vi "OutputShooter.vi"() -> ()   [LabVIEW 2020]
doc: "Runs feedback and feedforward control loops, manages safety interlocks, and sends commands to actuators specific to the shooter subsystem, specifically the lower shooter Falcon 500, the upper shooter Falcon 500, and the cowl Falcon 500."
uses:
  <vilib>/Rock Robotics/WPI/ThirdParty/Phoenix-LabVIEW/Motor Controller/Controls/CTRE_Phoenix_MotorControl_ControlMode.ctl
  60a0c6b8-2381-40aa-8ec2-a2ed4196b17e.vi
  0f04a1d6-f6ee-4c5b-8505-751c5889a14e.vi
  ceb5ace5-ff86-47da-bc92-28042f34dd1c.vi
  refnumbers.vi
  GRNF_CTREMotor.vi
  <vilib>/Rock Robotics/WPI/ThirdParty/Phoenix-LabVIEW/Motor Controller/Get/CTRE_Phoenix_MotorController_GetGeneralStatus.vi
  sensordata.vi
  robotconstants.vi
  robotoutputs.vi
  driverdata.vi
  drivercommands.vi
  TAI_Motor.vi
  <vilib>/Rock Robotics/WPI/ThirdParty/Phoenix-LabVIEW/Motor Controller/Get/CTRE_Phoenix_MotorController_GetSelectedSensorData.vi
  <vilib>/Rock Robotics/WPI/ThirdParty/Phoenix-LabVIEW/Motor Controller/Get/CTRE_Phoenix_MotorController_GetVoltage.vi
panel:
  in  "Shooter Upper PID Configuration":T1={"P Gain"=0.006, "I Gain"=0.0, "D Gain"=0.0, "F Gain"=0.2, "I Zone"=200.0} {"I Zone" step=0.01; "F Gain" step=0.01; "D Gain" step=0.01; "I Gain" step=0.01; "P Gain" min=0.0 step=0.01}
  out "Cowl Velocity":cluster{dbl}(graph)
  in  "Cowl PID Parameters":T2={"Kp"=0.03, "Ki"=0.0, "Kd"=0.0, "Kf (don't use)"=0.0, "I-Zone"=10.0} {"Kd" min=0.0; "Ki" min=0.0; "Kp" min=0.0}
  in  "Arbitrary Feed Forward [-1,1]":dbl=0.03
  in  "Cowl S-Curve Strength":i32=4
  in  "Cowl Acceleration (deg/s^2)":dbl=300.0
  in  "Cowl Cruise Velocity (deg/s)":dbl=60.0
  out "Cowl Position":cluster{dbl, "Interlock Output":dbl}(graph)
  out "Position":dbl
  in  "Plot Cowl":bool
  in  "Manual Override Cowl":bool
  in  "Manual Cowl Command (deg)":dbl
  in  "Manual Shooter Upper Speed Ratio":dbl=1.5 min=0.0 max=6000.0 step=100.0
  in  "Manual Shooter Speed Goal (rpm)":dbl min=0.0 max=6000.0 step=100.0
  in  "Override Shooter State Controller":bool
  out "Shooter Upper":T3(graph)
  in  "Plot Shooter":bool
  out "Shooter Lower":T3(graph)
  in  "Shooter Lower PID Configuration":T1={"P Gain"=0.005, "I Gain"=0.0, "D Gain"=0.0, "F Gain"=0.2, "I Zone"=200.0} {"I Zone" step=0.01; "F Gain" step=0.01; "D Gain" step=0.01; "I Gain" step=0.01; "P Gain" min=0.0 step=0.01}
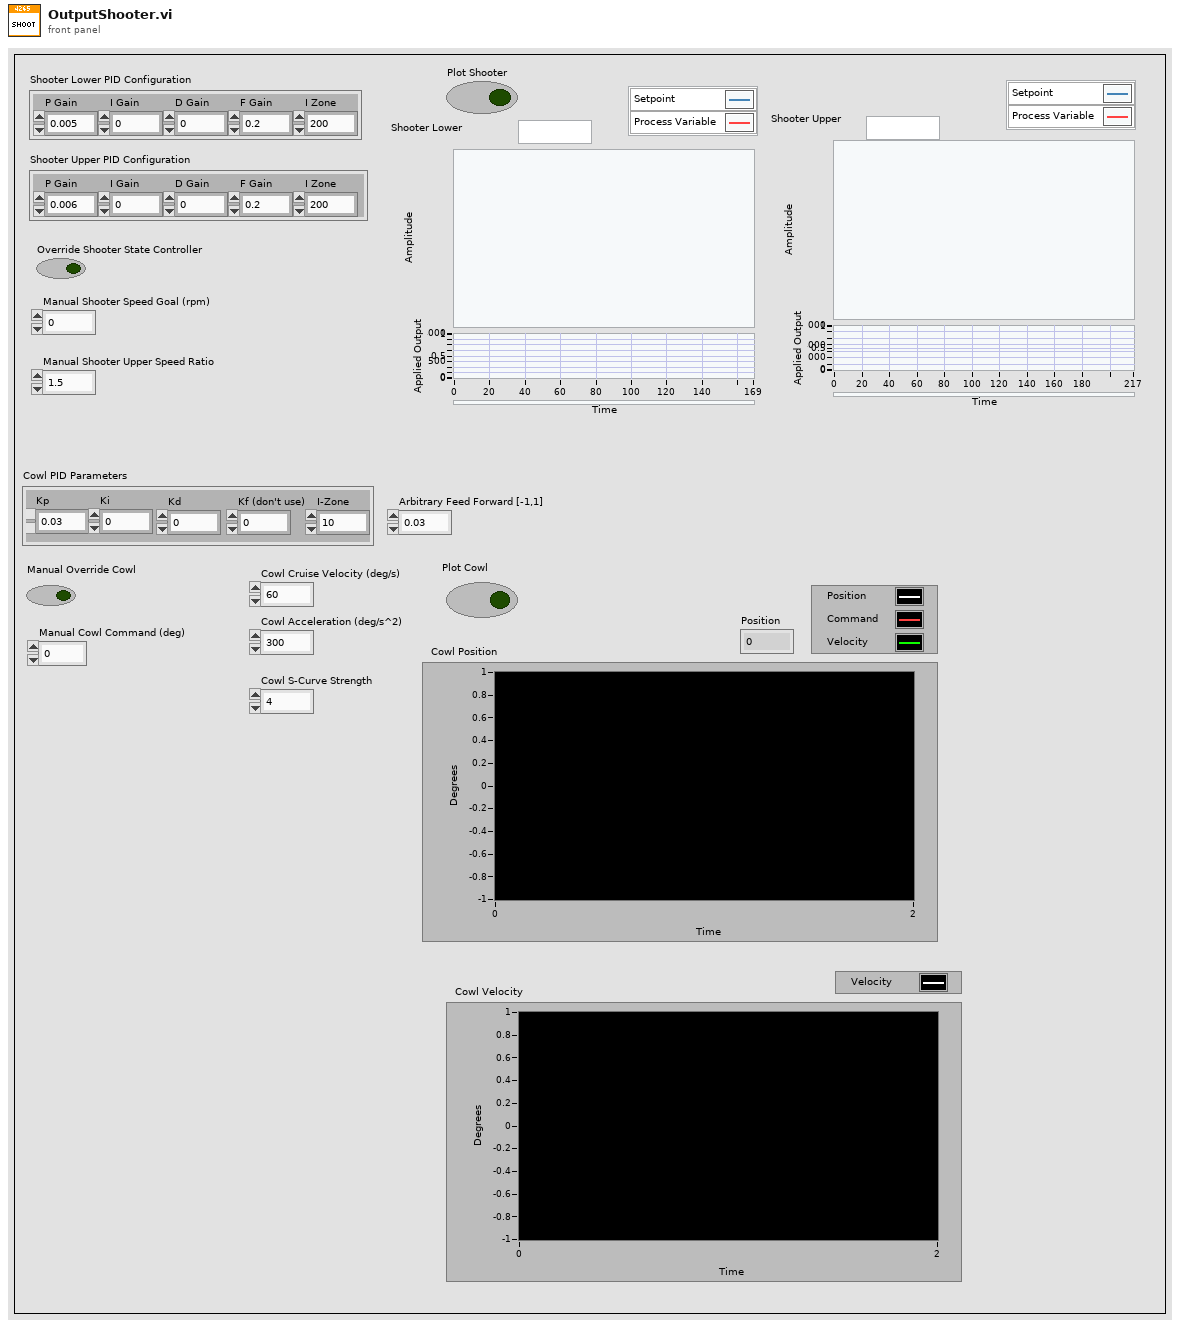
[diagram p1: front panel]
types:
  T1 = cluster{"P Gain":dbl, "I Gain":dbl, "D Gain":dbl, "F Gain":dbl, "I Zone":dbl}
  T2 = cluster{"Kp":dbl, "Ki":dbl, "Kd":dbl, "Kf (don't use)":dbl, "I-Zone":dbl}
  T3 = cluster{"Sensor Velocity":dbl, "Setpoint":dbl, "Applied Output":dbl}
  T4 = cluster{"Cowl Cruise Velocity (deg/s)":i32, "Cowl Acceleration (deg/s^2)":i32, "Cowl S-Curve Strength":i32}
  T5 = typedef "WPI_MotorControlDeviceRef.ctl" = cluster{"DeviceStatus":errorcluster, "Type":T6, "PWM":cluster{"PWM Channel":T7, "DeadBand":T8}, "CAN":cluster{"Device Number":u8, "SetOutput VI Ref":variant, "GetOutput VI Ref":variant, "Enable VI Ref":variant, "Disable VI Ref":variant, "Data":variant}, "Invert":bool, "DIO PWM":cluster{"PWM \"Enable\" Channel":T7, "DIOChannel":T9, "PWM Rate":dbl}}
  T6 = typedef "WPI_MotorControlType.ctl" = enum16{"PWM", "CAN", "DIO PWM"}
  T7 = typedef "FPGA_DIOPWMChannel.ctl" = enum8{"PWM 0", "PWM 1", "PWM 2", "PWM 3", "PWM 4", "PWM 5", "PWM 6", "PWM 7", "PWM 8", "PWM 9", "PWM MXP 0", "PWM MXP 1", "PWM MXP 2", "PWM MXP 3", "PWM MXP 4", "PWM MXP 5", "PWM MXP 6", "PWM MXP 7", "PWM MXP 8", "PWM MXP 9", "Invalid"}
  T8 = typedef "WPI_PWMDeadband.ctl" = cluster{"Name":string, "maxPositivePwm":i32, "minPositivePwm":i32, "centerPwm":i32, "maxNegativePwm":i32, "minNegativePwm":i32, "angularRange":u16}
  T9 = typedef "FPGA_DIOChannel.ctl" = enum8{"DIO 0", "DIO 1", "DIO 2", "DIO 3", "DIO 4", "DIO 5", "DIO 6", "DIO 7", "DIO 8", "DIO 9", "DIO MXP 0", "DIO MXP 1", "DIO MXP 2", "DIO MXP 3", "DIO MXP 4", "DIO MXP 5", "DIO MXP 6", "DIO MXP 7", "DIO MXP 8", "DIO MXP 9", "DIO MXP 10", "DIO MXP 11", "DIO MXP 12", "DIO MXP 13", "DIO MXP 14", "DIO MXP 15", "SPI Port CS1", "SPI Port CS2", "SPI Port CS3", "SPI Port MISO", "SPI Port MOSI", "Invalid"}
  T10 = cluster{"P Gain":bool, "I Gain":bool, "D Gain":bool, "F Gain":bool, "I Zone":bool}
  T11 = cluster{"Cowl Cruise Velocity (deg/s)":bool, "Cowl Acceleration (deg/s^2)":bool, "Cowl S-Curve Strength":bool}
  T12 = enum16{"No Changed Output", "New Normal Output", "New Testing Output"}
  T13 = cluster{"Kp":bool, "Ki":bool, "Kd":bool, "Kf (don't use)":bool, "I-Zone":bool}
  T14 = typedef "CTRE_Phoenix_MotorControl_ControlMode.ctl" = u16
  T15 = cluster{"Interlocked Output":dbl, dbl, "Percent Output":dbl}
  T16 = enum16{"DemandType_Neutral", "DemandType_AuxPID", "DemandType_ArbitraryFeedForward"}
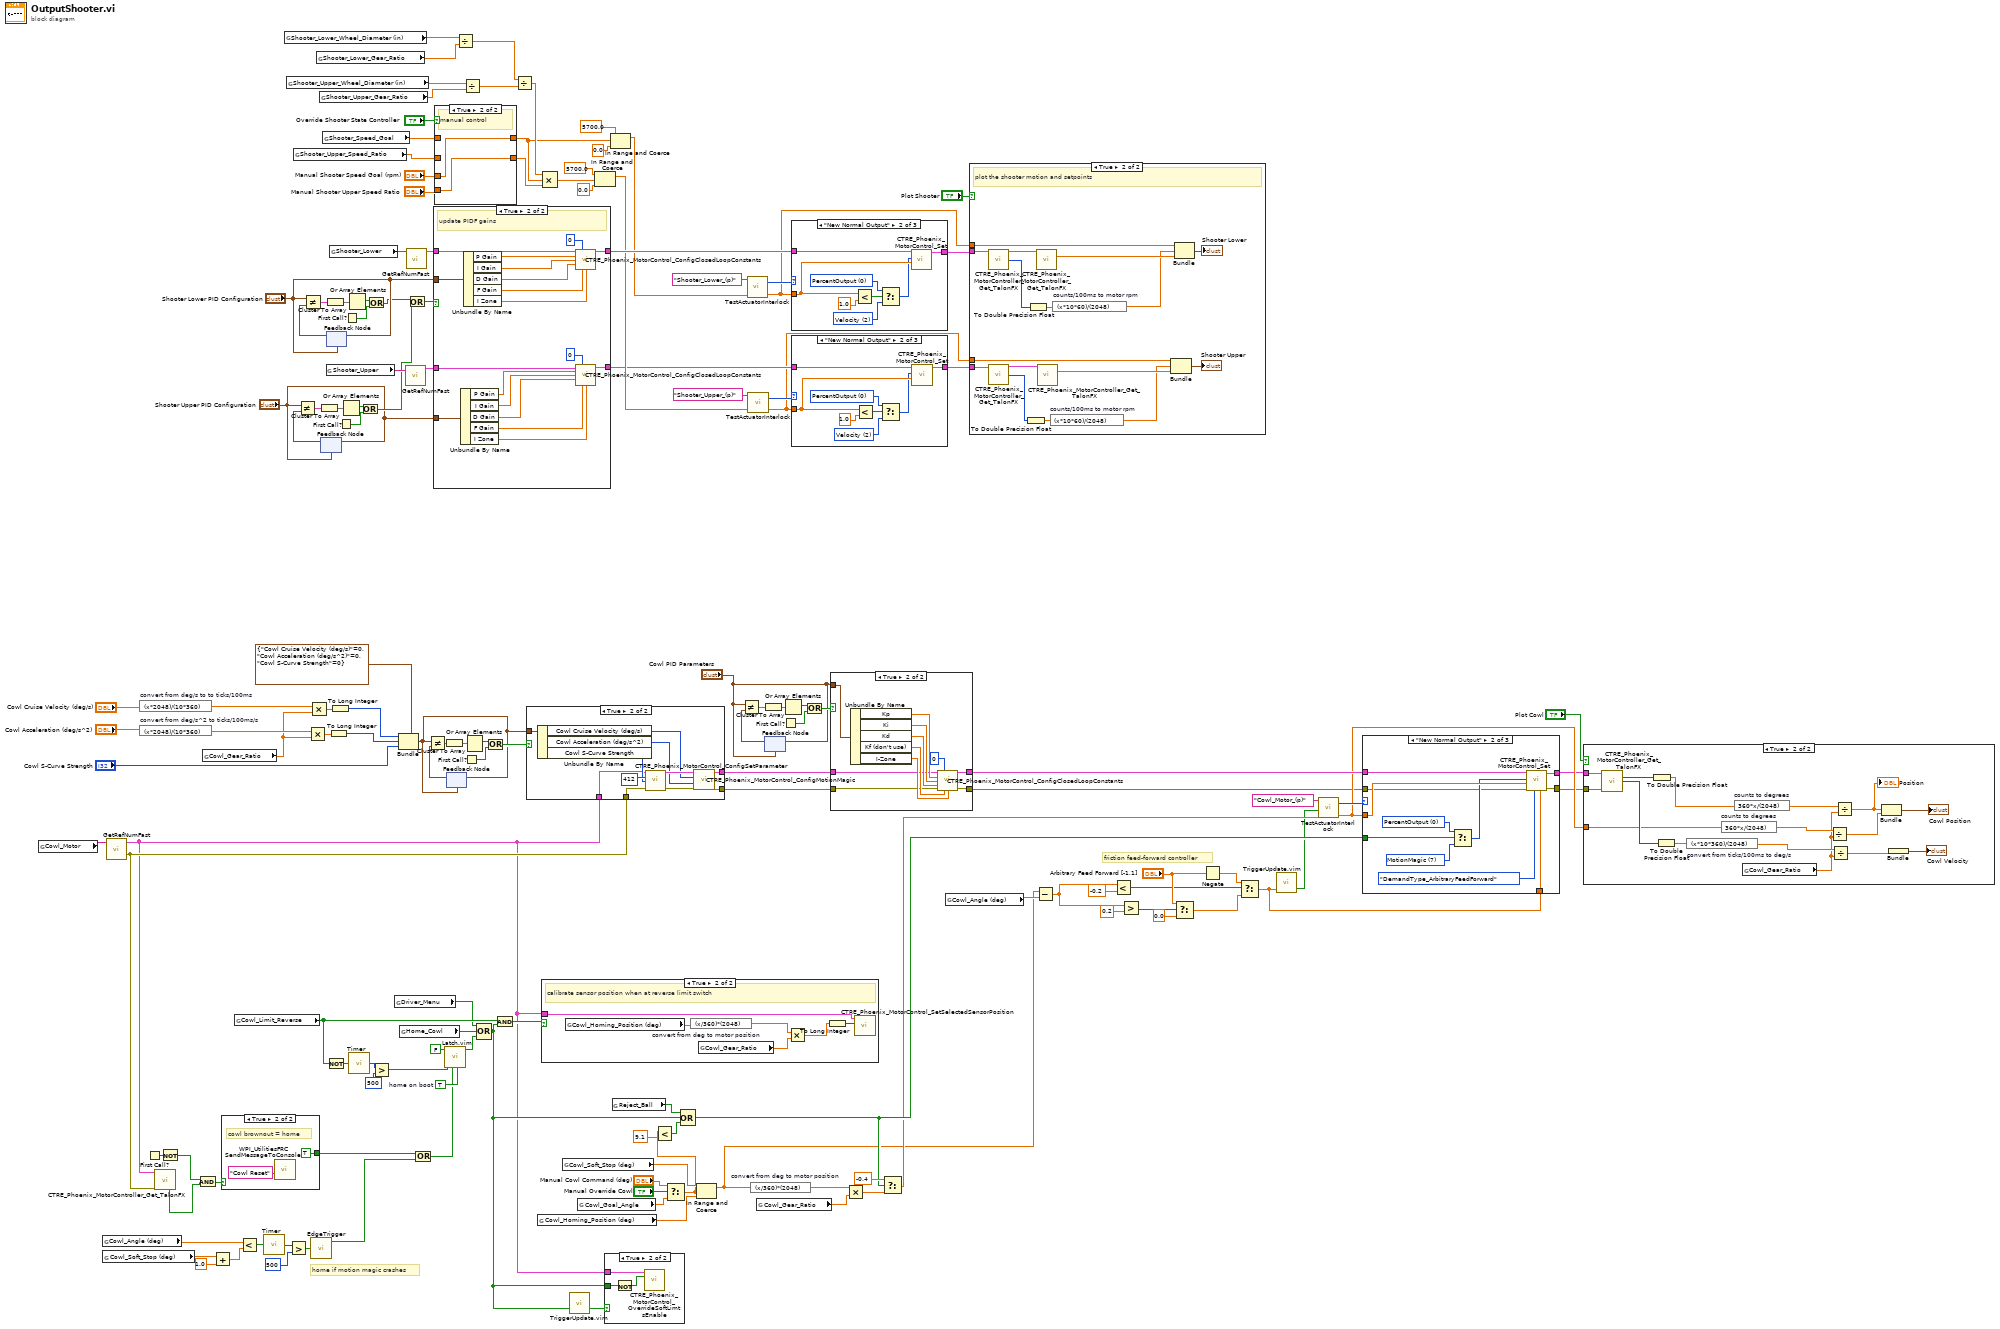
[diagram p0: block diagram]
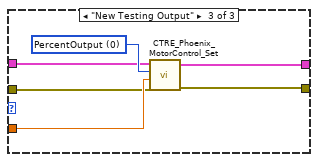
[diagram p4: hidden frame]
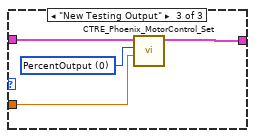
[diagram p6: hidden frame]
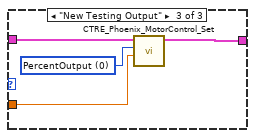
[diagram p8: hidden frame]
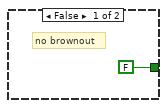
[diagram p9: hidden frame]
diagram:
  w29 = TRUE  # home on boot
  # "home if motion magic crashes"
  # "friction feed-forward controller"
  n1 = global read "refnumbers.vi" "Cowl_Motor"() -> (w129:string)
  n2 = global read "sensordata.vi" "Cowl_Angle (deg)"() -> (w7:dbl)
  n3 = global read "robotconstants.vi" "Cowl_Soft_Stop (deg)"() -> (w12:dbl)
  n4 = call-poly "GetRefNumFast.vi"("RefNum Name"=w129) -> ("Error"=w77:errorcluster, "Device Reference"=w9:T5)  [unwired: 5 in]
  n5 = expression code="(x*2048)/(10*360)" "convert from deg/s to to ticks/100ms"("Cowl Cruise Velocity (deg/s)") -> (w70:dbl)
  n6 = expression code="(x*2048)/(10*360)" "convert from deg/s^2 to ticks/100ms/s"("Cowl Acceleration (deg/s^2)") -> (w71:dbl)
  n7 = First Call?() -> (First Call?: T/F=w99:bool)
  n8 = call-poly <vilib>:"CTRE_Phoenix_MotorController_Get_TalonFX.vi"("PhoenixMotorControlDevRef"=w9, "error in"=w77) -> ("Has Reset Occurred?"=w97:bool)  [unwired: 8 in, 5 out]
  n9 = Not(x=w99) -> (.not. x?=w98:bool)
  n10 = And(x=w98, y=w97) -> (x .and. y?=w100:bool)
  n11 = global read "robotconstants.vi" "Cowl_Gear_Ratio"() -> (w69:dbl)
  n12 = Add(x=w12, y=1.0) -> (x+y=w6:dbl)
  n13 = case shown="True" w100 {
    tunnel: [FALSE TRUE] -> w16
    frame False {
      # "no brownout"
    }
    frame True {
      # "cowl brownout = home"
      n14 = call <vilib>:"WPI_UtilitiesFRC SendMessageToConsole.vi"("Message"="Cowl Reset") -> ()  [unwired: 14 in, 1 out]
    }
  }
  n15 = global read "sensordata.vi" "Cowl_Limit_Reverse"() -> (w26:bool)
  n16 = Less?(x=w7, y=w6) -> (x < y?=w5:bool)
  n17 = call "Timer.vi"("Reset Timer"=w5) -> ("Time (ms)"=w17:u32)
  n18 = global read "robotconstants.vi" "Shooter_Lower_Wheel_Diameter (in)"() -> (w40:dbl)
  n19 = global read "robotconstants.vi" "Shooter_Upper_Wheel_Diameter (in)"() -> (w37:dbl)
  n20 = Greater?(x=w17, y=u32 500) -> (0:w14:bool)
  n21 = global read "robotoutputs.vi" "Shooter_Upper_Speed_Ratio"() -> (w107:dbl)
  n22 = Multiply(x=w71, y=w69) -> (x*y=w72:dbl)
  n23 = Multiply(x=w70, y=w69) -> (x*y=w73:dbl)
  n24 = call "EdgeTrigger.vi"("Input Signal"=w14) -> ("Rising Edge Trigger"=w13:bool)  [unwired: 2 out]
  n25 = global read "robotconstants.vi" "Shooter_Lower_Gear_Ratio"() -> (w39:dbl)
  n26 = global read "robotconstants.vi" "Shooter_Upper_Gear_Ratio"() -> (w36:dbl)
  n27 = feedback #1("Shooter Upper PID Configuration") -> (w45:T1)
  n28 = Not Equal?(x="Shooter Upper PID Configuration", y=w45) -> (x != y?=w47:T10)
  n29 = Cluster To Array(cluster=w47) -> (array=w46:bool[])
  n30 = feedback-in #1("Shooter Upper PID Configuration") -> ()
  n31 = global read "robotoutputs.vi" "Shooter_Speed_Goal"() -> (w108:dbl)
  n32 = global read "refnumbers.vi" "Shooter_Upper"() -> (w135:string)
  n33 = Not(x=w26) -> (.not. x?=w28:bool)
  n34 = feedback #2("Shooter Lower PID Configuration") -> (w141:T1)
  n35 = Not Equal?(x="Shooter Lower PID Configuration", y=w141) -> (x != y?=w143:T10)
  n36 = Cluster To Array(cluster=w143) -> (array=w142:bool[])
  n37 = feedback-in #2("Shooter Lower PID Configuration") -> ()
  n38 = To Long Integer(number=w72) -> (32bit integer=w64:i32)
  n39 = global read "refnumbers.vi" "Shooter_Lower"() -> (w136:string)
  n40 = To Long Integer(number=w73) -> (32bit integer=w65:i32)
  n41 = First Call?() -> (First Call?: T/F=w49:bool)
  n42 = Or Array Elements(Boolean array=w46) -> (logical OR=w48:bool)
  n43 = First Call?() -> (First Call?: T/F=w145:bool)
  n44 = Or Array Elements(Boolean array=w142) -> (logical OR=w144:bool)
  n45 = call "Timer.vi"("Reset Timer"=w28) -> ("Time (ms)"=w32:u32)
  n46 = Or(x=w48, y=w49) -> (x .or. y?=w42:bool)
  n47 = Or(x=w144, y=w145) -> (x .or. y?=w43:bool)
  n48 = Greater?(x=w32, y=u32 500) -> (0:w27:bool)
  n49 = global read "drivercommands.vi" "Driver_Menu"() -> (w1:bool)
  n50 = Bundle(cluster=T4 {"Cowl Cruise Velocity (deg/s)"=0, "Cowl Acceleration (deg/s^2)"=0, "Cowl S-Curve Strength"=0}, "Cowl Cruise Velocity (deg/s)"=w65, "Cowl Acceleration (deg/s^2)"=w64, "Cowl S-Curve Strength"="Cowl S-Curve Strength") -> (w110:T4)
  n51 = global read "driverdata.vi" "Home_Cowl"() -> (w22:bool)
  n52 = call-poly "GetRefNumFast.vi"("RefNum Name"=w135) -> ("Device Reference"=w138:T5)  [unwired: 5 in, 1 out]
  n53 = call-poly "GetRefNumFast.vi"("RefNum Name"=w136) -> ("Device Reference"=w140:T5)  [unwired: 5 in, 1 out]
  n54 = Or(x=w43, y=w42) -> (x .or. y?=w44:bool)
  n55 = Compound Arithmetic op=OR(w16, w13) -> (w15:bool)
  n56 = case shown="True" w44 {
    tunnel: w140 -> [w150 w167]
    tunnel: "Shooter Lower PID Configuration" -> [_ w166]
    tunnel: [w150 w168] -> w94
    tunnel: [w149 w165] -> w87
    tunnel: w138 -> [w149 w164]
    tunnel: "Shooter Upper PID Configuration" -> [_ w156]
    frame False {
      # "do not update PIDF gains"
    }
    frame True {
      # "update PIDF gains"
      n57 = Unbundle By Name(w156) -> ("P Gain"=w155:dbl, "I Gain"=w154:dbl, "D Gain"=w153:dbl, "F Gain"=w152:dbl, "I Zone"=w151:dbl)
      n58 = Unbundle By Name(w166) -> ("P Gain"=w163:dbl, "I Gain"=w162:dbl, "D Gain"=w161:dbl, "F Gain"=w157:dbl, "I Zone"=w160:dbl)
      n59 = call <vilib>:"CTRE_Phoenix_MotorControl_ConfigClosedLoopConstants.vi"("PhoenixMotorControlDevRef"=w167, "slotIdx"=0, "P"=w163, "I"=w162, "D"=w161, "F"=w157, "I Zone"=w160) -> ("PhoenixMotorControlDevRef"=w168:T5)  [unwired: 7 in, 1 out]
      n60 = call <vilib>:"CTRE_Phoenix_MotorControl_ConfigClosedLoopConstants.vi"("PhoenixMotorControlDevRef"=w164, "slotIdx"=0, "P"=w155, "I"=w154, "D"=w153, "F"=w152, "I Zone"=w151) -> ("PhoenixMotorControlDevRef"=w165:T5)  [unwired: 7 in, 1 out]
    }
  }
  n61 = case shown="True" "Override Shooter State Controller" {
    tunnel: "Manual Shooter Speed Goal (rpm)" -> [_ w172]
    tunnel: "Manual Shooter Upper Speed Ratio" -> [_ w171]
    tunnel: w107 -> [w169 _]
    tunnel: w108 -> [w170 _]
    tunnel: [w170 w172] -> w104
    tunnel: [w169 w171] -> w131
    frame False {
      # "state controller"
    }
    frame True {
      # "manual control"
    }
  }
  n62 = call "Latch.vim"("Default Value"=w29, "Reset"=w15, "Latch Signal"=w27, "Latch Value"=FALSE) -> ("Latched"=w25:bool)  [unwired: 7 in]
  n63 = feedback #3(w110) -> (w111:T4)
  n64 = Not Equal?(x=w110, y=w111) -> (x != y?=w114:T11)
  n65 = Cluster To Array(cluster=w114) -> (array=w113:bool[])
  n66 = feedback-in #3(w110) -> ()
  n67 = Divide(x=w40, y=w39) -> (x/y=w38:dbl)
  n68 = First Call?() -> (First Call?: T/F=w116:bool)
  n69 = Divide(x=w37, y=w36) -> (x/y=w35:dbl)
  n70 = Or Array Elements(Boolean array=w113) -> (logical OR=w115:bool)
  n71 = Compound Arithmetic op=OR(w1, w22, w25) -> (w10:bool)
  n72 = Or(x=w115, y=w116) -> (x .or. y?=w112:bool)
  n73 = And(x=w26, y=w10) -> (x .and. y?=w23:bool)
  n74 = Divide(x=w38, y=w35) -> (x/y=w130:dbl)
  n75 = case shown="True" w112 {
    tunnel: w110 -> [_ w182]
    tunnel: w9 -> [w174 w178]
    tunnel: w77 -> [w173 w177]
    tunnel: [w174 w176] -> w84
    tunnel: [w173 w175] -> w83
    frame False {
    }
    frame True {
      n76 = Unbundle By Name(w182) -> ("Cowl Cruise Velocity (deg/s)"=w179:i32, "Cowl Acceleration (deg/s^2)"=w180:i32, "Cowl S-Curve Strength"=w181:i32)
      n77 = call <vilib>:"CTRE_Phoenix_MotorControl_ConfigSetParameter.vi"("PhoenixMotorControlDevRef"=w178, "Parameter"=412 ("New Sensor Position"), "value"=w181, "error in (no error)"=w177) -> ("PhoenixMotorControlDevRef"=w184:T5, "error out"=w183:errorcluster)  [unwired: 10 in]
      n78 = call <vilib>:"CTRE_Phoenix_MotorControl_ConfigMotionMagic.vi"("error in (no error)"=w183, "Acceleration"=w180, "Cruise Velocity"=w179, "PhoenixMotorControlDevRef"=w184) -> ("error out"=w175:errorcluster, "PhoenixMotorControlDevRef"=w176:T5)  [unwired: 6 in]
    }
  }
  n79 = global read "robotconstants.vi" "Cowl_Homing_Position (deg)"() -> (w19:dbl)
  n80 = case shown="True" w23 {
    tunnel: w9 -> [_ w190]
    frame False {
    }
    frame True {
      # "calibrate sensor position when at reverse limit switch"
      n81 = global read "robotconstants.vi" "Cowl_Homing_Position (deg)"() -> (w189:dbl)
      n82 = expression code="(x/360)*(2048)" "convert from deg to motor position"(w189) -> (w187:dbl)
      n83 = global read "robotconstants.vi" "Cowl_Gear_Ratio"() -> (w188:dbl)
      n84 = Multiply(x=w187, y=w188) -> (x*y=w186:dbl)
      n85 = To Long Integer(number=w186) -> (32bit integer=w191:i32)
      n86 = call <vilib>:"CTRE_Phoenix_MotorControl_SetSelectedSensorPosition.vi"("New Sensor Position"=w191, "PhoenixMotorControlDevRef"=w190) -> ()  [unwired: 8 in, 2 out]
    }
  }
  n87 = Compound Arithmetic op=MULTIPLY(w130, w104, w131) -> (w101:dbl)
  n88 = global read "robotconstants.vi" "Cowl_Soft_Stop (deg)"() -> (w52:dbl)
  n89 = call "TriggerUpdate.vim"("Trigger"=w10) -> ("Update"=w11:bool)  [unwired: 2 in]
  n90 = global read "robotoutputs.vi" "Cowl_Goal_Angle"() -> (w109:dbl)
  n91 = In Range and Coerce(upper limit=5700.0, x=w101, lower limit=0.0) -> (coerced(x)=w88:dbl)  [unwired: 1 out]
  n92 = case shown="True" w11 {
    tunnel: w10 -> [_ w194]
    tunnel: w9 -> [_ w192]
    frame False {
    }
    frame True {
      n93 = Not(x=w194) -> (.not. x?=w193:bool)
      n94 = call <vilib>:"CTRE_Phoenix_MotorControl_OverrideSoftLimtsEnable.vi"("PhoenixMotorControlDevRef"=w192, "Override Soft Limit Enable?"=w193) -> ()  [unwired: 12 in, 2 out]
    }
  }
  n95 = In Range and Coerce(upper limit=5700.0, x=w104, lower limit=0.0) -> (coerced(x)=w93:dbl)  [unwired: 1 out]
  n96 = global read "robotoutputs.vi" "Reject_Ball"() -> (w24:bool)
  n97 = Select(t="Manual Cowl Command (deg)", s="Manual Override Cowl", f=w109) -> (s? t:f=w3:dbl)
  n98 = Less?(x=w3, y=9.1) -> (x < y?=w4:bool)
  n99 = Compound Arithmetic op=OR(w24, w10, w4) -> (w79:bool)
  n100 = In Range and Coerce(upper limit=w52, x=w3, lower limit=w19) -> (coerced(x)=w50:dbl)  [unwired: 1 out]
  n101 = call-poly "TestActuatorInterlock.vi"("Normal Output"=w93, "Actuator Name"="Shooter_Lower_(p)" ("Actuator_Name")) -> ("Interlocked Output"=w92:dbl, "Output Mode"=w96:T12)  [unwired: 3 in]
  n102 = call-poly "TestActuatorInterlock.vi"("Normal Output"=w88, "Actuator Name"="Shooter_Upper_(p)" ("Actuator_Name")) -> ("Interlocked Output"=w85:dbl, "Output Mode"=w90:T12)  [unwired: 3 in]
  n103 = expression code="(x/360)*(2048)" "convert from deg to motor position"(w50) -> (w74:dbl)
  n104 = global read "robotconstants.vi" "Cowl_Gear_Ratio"() -> (w75:dbl)
  n105 = feedback #4("Cowl PID Parameters") -> (w119:T2)
  n106 = Not Equal?(x="Cowl PID Parameters", y=w119) -> (x != y?=w122:T13)
  n107 = Cluster To Array(cluster=w122) -> (array=w121:bool[])
  n108 = feedback-in #4("Cowl PID Parameters") -> ()
  n109 = First Call?() -> (First Call?: T/F=w124:bool)
  n110 = Or Array Elements(Boolean array=w121) -> (logical OR=w123:bool)
  n111 = case shown="\"New Normal Output\"" w96 {
    tunnel: w94 -> [w195 w203 w206]
    tunnel: w92 -> [_ w198 w205]
    tunnel: [w195 w202 w204] -> w91
    frame "No Changed Output", Default {
    }
    frame "New Normal Output" {
      w200 = T14 0 items=["PercentOutput"=0, "Position"=1, "Velocity"=2, "Current"=3, "Follower"=5, "MotionProfile"=6, "MotionMagic"=7, "MotionProfileArc"=10, "Disabled"=15] ("Control Mode")
      w201 = T14 2 items=["PercentOutput"=0, "Position"=1, "Velocity"=2, "Current"=3, "Follower"=5, "MotionProfile"=6, "MotionMagic"=7, "MotionProfileArc"=10, "Disabled"=15] ("Control Mode")
      n112 = Less?(x=w198, y=1.0) -> (x < y?=w197:bool)
      n113 = Select(t=w200, s=w197, f=w201) -> (s? t:f=w196:T14)
      n114 = call <vilib>:"CTRE_Phoenix_MotorControl_Set.vi"("Output"=w198, "Control Mode"=w196, "PhoenixMotorControlDevRef"=w203) -> ("PhoenixMotorControlDevRef"=w202:T5)  [unwired: 7 in, 1 out]
    }
    frame "New Testing Output" {
      w207 = T14 0 items=["PercentOutput"=0, "Position"=1, "Velocity"=2, "Current"=3, "Follower"=5, "MotionProfile"=6, "MotionMagic"=7, "MotionProfileArc"=10, "Disabled"=15] ("Control Mode")
      n115 = call <vilib>:"CTRE_Phoenix_MotorControl_Set.vi"("Output"=w205, "Control Mode"=w207, "PhoenixMotorControlDevRef"=w206) -> ("PhoenixMotorControlDevRef"=w204:T5)  [unwired: 7 in, 1 out]
    }
  }
  n116 = case shown="\"New Normal Output\"" w90 {
    tunnel: w87 -> [w208 w216 w219]
    tunnel: w85 -> [_ w211 w218]
    tunnel: [w208 w215 w217] -> w86
    frame "No Changed Output", Default {
    }
    frame "New Normal Output" {
      w213 = T14 0 items=["PercentOutput"=0, "Position"=1, "Velocity"=2, "Current"=3, "Follower"=5, "MotionProfile"=6, "MotionMagic"=7, "MotionProfileArc"=10, "Disabled"=15] ("Control Mode")
      w214 = T14 2 items=["PercentOutput"=0, "Position"=1, "Velocity"=2, "Current"=3, "Follower"=5, "MotionProfile"=6, "MotionMagic"=7, "MotionProfileArc"=10, "Disabled"=15] ("Control Mode")
      n117 = Less?(x=w211, y=1.0) -> (x < y?=w210:bool)
      n118 = Select(t=w213, s=w210, f=w214) -> (s? t:f=w209:T14)
      n119 = call <vilib>:"CTRE_Phoenix_MotorControl_Set.vi"("Output"=w211, "Control Mode"=w209, "PhoenixMotorControlDevRef"=w216) -> ("PhoenixMotorControlDevRef"=w215:T5)  [unwired: 7 in, 1 out]
    }
    frame "New Testing Output" {
      w220 = T14 0 items=["PercentOutput"=0, "Position"=1, "Velocity"=2, "Current"=3, "Follower"=5, "MotionProfile"=6, "MotionMagic"=7, "MotionProfileArc"=10, "Disabled"=15] ("Control Mode")
      n120 = call <vilib>:"CTRE_Phoenix_MotorControl_Set.vi"("Output"=w218, "Control Mode"=w220, "PhoenixMotorControlDevRef"=w219) -> ("PhoenixMotorControlDevRef"=w217:T5)  [unwired: 7 in, 1 out]
    }
  }
  n121 = Or(x=w123, y=w124) -> (x .or. y?=w120:bool)
  n122 = case shown="True" w120 {
    tunnel: "Cowl PID Parameters" -> [_ w229]
    tunnel: w84 -> [w222 w226]
    tunnel: w83 -> [w221 w225]
    tunnel: [w222 w224] -> w80
    tunnel: [w221 w223] -> w76
    frame False {
    }
    frame True {
      n123 = Unbundle By Name(w229) -> ("Kp"=w231:dbl, "Ki"=w232:dbl, "Kd"=w233:dbl, "Kf (don't use)"=w228:dbl, "I-Zone"=w227:dbl)
      n124 = call <vilib>:"CTRE_Phoenix_MotorControl_ConfigClosedLoopConstants.vi"("PhoenixMotorControlDevRef"=w226, "slotIdx"=0, "P"=w231, "I"=w232, "D"=w233, "error in (no error)"=w225, "F"=w228, "I Zone"=w227) -> ("PhoenixMotorControlDevRef"=w224:T5, "error out"=w223:errorcluster)  [unwired: 6 in]
    }
  }
  n125 = Multiply(x=w74, y=w75) -> (x*y=w51:dbl)
  n126 = Select(t=-0.4, s=w79, f=w51) -> (s? t:f=w63:dbl)
  n127 = global read "sensordata.vi" "Cowl_Angle (deg)"() -> (w62:dbl)
  n128 = case shown="True" "Plot Shooter" {
    tunnel: w92 -> [_ w249]
    tunnel: w91 -> [_ w245]
    tunnel: w86 -> [_ w244]
    tunnel: w85 -> [_ w242]
    frame False {
      # "disable plotting and expensive sensor polling"
    }
    frame True {
      # "plot the shooter motion and setpoints"
      n129 = call-poly <vilib>:"CTRE_Phoenix_MotorController_Get_TalonFX.vi"("PhoenixMotorControlDevRef"=w245) -> ("PhoenixMotorControlDevRef"=w246:T5, "Velocity (Raw Sensor Units per 100 ms)"=w240:i32)  [unwired: 11 in, 2 out]
      n130 = call-poly <vilib>:"CTRE_Phoenix_MotorController_Get_TalonFX.vi"("PhoenixMotorControlDevRef"=w244) -> ("PhoenixMotorControlDevRef"=w243:T5, "Velocity (Raw Sensor Units per 100 ms)"=w235:i32)  [unwired: 11 in, 2 out]
      n131 = To Double Precision Float(number=w235) -> (double precision float=w236:dbl)
      n132 = To Double Precision Float(number=w240) -> (double precision float=w241:dbl)
      n133 = call-poly <vilib>:"CTRE_Phoenix_MotorController_Get_TalonFX.vi"("PhoenixMotorControlDevRef"=w246) -> ("Percent Output"=w247:dbl)  [unwired: 10 in, 4 out]
      n134 = call-poly <vilib>:"CTRE_Phoenix_MotorController_Get_TalonFX.vi"("PhoenixMotorControlDevRef"=w243) -> ("Percent Output"=w248:dbl)  [unwired: 10 in, 4 out]
      n135 = expression code="(x*10*60)/(2048)" "counts/100ms to motor rpm"(w236) -> (w234:dbl)
      n136 = expression code="(x*10*60)/(2048)" "counts/100ms to motor rpm"(w241) -> (w239:dbl)
      n137 = Bundle("Interlocked Output"=w242, w234, "Percent Output"=w248) -> (→"Shooter Upper":T15)  [unwired: 1 in]
      n138 = Bundle("Interlocked Output"=w249, w239, "Percent Output"=w247) -> (→"Shooter Lower":T15)  [unwired: 1 in]
    }
  }
  n139 = Subtract(x=w50, y=w62) -> (x-y=w56:dbl)
  n140 = Less?(x=w56, y=-0.2) -> (x < y?=w53:bool)
  n141 = Greater?(x=w56, y=0.2) -> (0:w61:bool)
  n142 = Select(t="Arbitrary Feed Forward [-1,1]", s=w61, f=0.0) -> (s? t:f=w60:dbl)
  n143 = Negate(x="Arbitrary Feed Forward [-1,1]") -> (-x=w59:dbl)
  n144 = Select(t=w59, s=w53, f=w60) -> (s? t:f=w33:dbl)
  n145 = call "TriggerUpdate.vim"("Trigger"=w33) -> ("Update"=w34:bool)  [unwired: 2 in]
  n146 = call-poly "TestActuatorInterlock.vi"("Normal Output"=w63, "Aux Trigger"=w34, "Actuator Name"="Cowl_Motor_(p)" ("Actuator_Name")) -> ("Interlocked Output"=w78:dbl, "Output Mode"=w82:T12)  [unwired: 2 in]
  n147 = case shown="\"New Normal Output\"" w82 {
    tunnel: w80 -> [w251 w262 w267]
    tunnel: w78 -> [_ w258 w266]
    tunnel: [w251 w261 w265] -> w21
    tunnel: w79 -> [_ w256 _]
    tunnel: w33 -> [_ w254 _]
    tunnel: [w250 w253 w263] -> w20
    tunnel: w76 -> [w250 w252 w264]
    frame "No Changed Output", Default {
    }
    frame "New Normal Output" {
      w259 = T14 0 items=["PercentOutput"=0, "Position"=1, "Velocity"=2, "Current"=3, "Follower"=5, "MotionProfile"=6, "MotionMagic"=7, "MotionProfileArc"=10, "Disabled"=15] ("Control Mode")
      w260 = T14 7 items=["PercentOutput"=0, "Position"=1, "Velocity"=2, "Current"=3, "Follower"=5, "MotionProfile"=6, "MotionMagic"=7, "MotionProfileArc"=10, "Disabled"=15] ("Control Mode")
      n148 = Select(t=w259, s=w256, f=w260) -> (s? t:f=w257:T14)
      n149 = call <vilib>:"CTRE_Phoenix_MotorControl_Set.vi"("Demand1"=w254, "DemandType"=T16."DemandType_ArbitraryFeedForward", "error in (no error)"=w252, "Output"=w258, "Control Mode"=w257, "PhoenixMotorControlDevRef"=w262) -> ("error out"=w253:errorcluster, "PhoenixMotorControlDevRef"=w261:T5)  [unwired: 4 in]
    }
    frame "New Testing Output" {
      w268 = T14 0 items=["PercentOutput"=0, "Position"=1, "Velocity"=2, "Current"=3, "Follower"=5, "MotionProfile"=6, "MotionMagic"=7, "MotionProfileArc"=10, "Disabled"=15] ("Control Mode")
      n150 = call <vilib>:"CTRE_Phoenix_MotorControl_Set.vi"("error in (no error)"=w264, "Output"=w266, "Control Mode"=w268, "PhoenixMotorControlDevRef"=w267) -> ("error out"=w263:errorcluster, "PhoenixMotorControlDevRef"=w265:T5)  [unwired: 6 in]
    }
  }
  n151 = case shown="True" "Plot Cowl" {
    tunnel: w78 -> [_ w277]
    tunnel: w20 -> [_ w280]
    tunnel: w21 -> [_ w279]
    frame False {
    }
    frame True {
      n152 = call-poly <vilib>:"CTRE_Phoenix_MotorController_Get_TalonFX.vi"("PhoenixMotorControlDevRef"=w279, "error in"=w280) -> ("Position (Raw Sensor Units)"=w282:i32, "Velocity (Raw Sensor Units per 100 ms)"=w283:i32)  [unwired: 10 in, 2 out]
      n153 = To Double Precision Float(number=w282) -> (double precision float=w281:dbl)
      n154 = To Double Precision Float(number=w283) -> (double precision float=w284:dbl)
      n155 = expression code="(x*10*360)/(2048)" "convert from ticks/100ms to deg/s"(w284) -> (w275:dbl)
      n156 = expression code="360*x/(2048)" "counts to degrees"(w277) -> (w273:dbl)
      n157 = expression code="360*x/(2048)" "counts to degrees"(w281) -> (w270:dbl)
      n158 = global read "robotconstants.vi" "Cowl_Gear_Ratio"() -> (w271:dbl)
      n159 = Divide(x=w273, y=w271) -> (x/y=w272:dbl)
      n160 = Divide(x=w275, y=w271) -> (x/y=w274:dbl)
      n161 = Divide(x=w270, y=w271) -> (x/y=w269:dbl)
      "Position" <- w269
      n162 = Bundle(w269, w272) -> (→"Cowl Position":cluster{dbl, dbl})  [unwired: 1 in]
      n163 = Bundle(w274) -> (→"Cowl Velocity":cluster{dbl})  [unwired: 1 in]
    }
  }
